vi "Configure Trace.vi"   [LabVIEW 2022 SP3, in "Agilent N934X Series.lvlib"]
doc: "This is a poly VI for configure trace."
uses:
  <instrlib>/Agilent N934X Series/Agilent N934X Series.lvlib
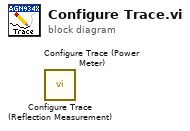
[diagram p0: block diagram]
diagram:
  n1 = call <instrlib>:"Configure Trace (Reflection Measurement).vi"() -> ()  [unwired: 10 in, 2 out]
  n2 = call <instrlib>:"Configure Trace (Power Meter).vi"() -> ()  [unwired: 10 in, 2 out]
